vi "Create (File).vi"(7 "Main Format":T1, 8 "error in (no error)":errorcluster, 9 "Main Filename":string, 10 "Config Root":path) -> (0 "error out":errorcluster, 3 "VolatusConfig out":refnum<class "VolatusConfig.lvclass">)   [LabVIEW 2020, in "VolatusConfig.lvlib" / "VolatusConfig.lvclass"]
uses:
  VolatusConfig.lvclass
  Config Format.ctl
  VolatusConfig.lvclass/VolatusConfig.ctl
  VolatusConfig.lvlib
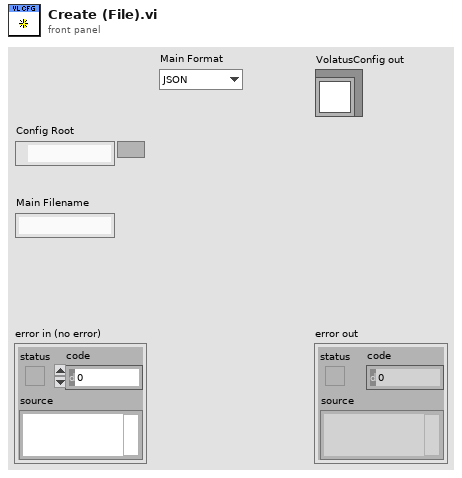
[diagram p1: front panel]
types:
  T1 = typedef "VolatusConfig.lvlib/Config Format.ctl" = enum16{"JSON", "INI", "SQLite"}
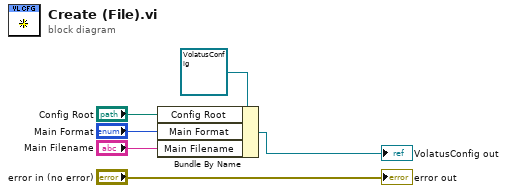
[diagram p0: block diagram]
diagram:
  n1 = Bundle By Name(cluster=refnum<class "VolatusConfig.lvclass"> refnum ("VolatusConfig in"), "Config Root"="Config Root", "Main Format"="Main Format", "Main Filename"="Main Filename") -> (→"VolatusConfig out":refnum<class "VolatusConfig.lvclass">)
  "error out" <- "error in (no error)"
